vi "Controller Generate Filter Coefficients From Transfer Function.vi"(0 "numerator":dbl[](array[numeric]), 1 "iwl coeff a":i16=2, 3 "iwl coeff b":i16=2, 5 "denominator":dbl[](array[numeric]), 9 "wl":i16=20, 11 "Generate FPGA Code?":bool, 12 "Filter Name":string, 14 "Destination Folder":path) -> (4 "coeff b":dbl[](array[numeric]), 6 "coeff a":dbl[](array[numeric]), 8 "gain":dbl)   [LabVIEW 2011, in "Controller VIs.lvlib"]
uses:
  Controller VIs.lvlib
  <vilib>/addons/Digital Filter Design/_Objects.llb/DFD Output Iwl Obj.ctl
  <vilib>/addons/Digital Filter Design/_Objects.llb/DFD Quantization Settings.ctl
  <vilib>/addons/Digital Filter Design/_Objects.llb/DFD Quantization Sources.ctl
  <vilib>/addons/Digital Filter Design/_Objects.llb/DFD Coef Norm Type.ctl
  <vilib>/addons/Digital Filter Design/_Objects.llb/DFD Phase Setting.ctl
  <vilib>/addons/Digital Filter Design/FXPModel.llb/DFD FXP Quantize Coef (Advanced).vi
  <vilib>/addons/Digital Filter Design/NI_DigFilterLicensed.lvlib
  <vilib>/addons/Digital Filter Design/CodeGen.llb/DFD FXP LabVIEW FPGA Code Generator.vi
panel:
  in  "Error Graph?":bool
  out "phase (deg)":cluster{"Y":dbl[], "Y":dbl[]}[](graph)
  out "gain (dB)":cluster{"Y":dbl[], "Y":dbl[]}[](graph)
  out "max gain error (dB)":dbl
  out "max phase error (deg)":dbl
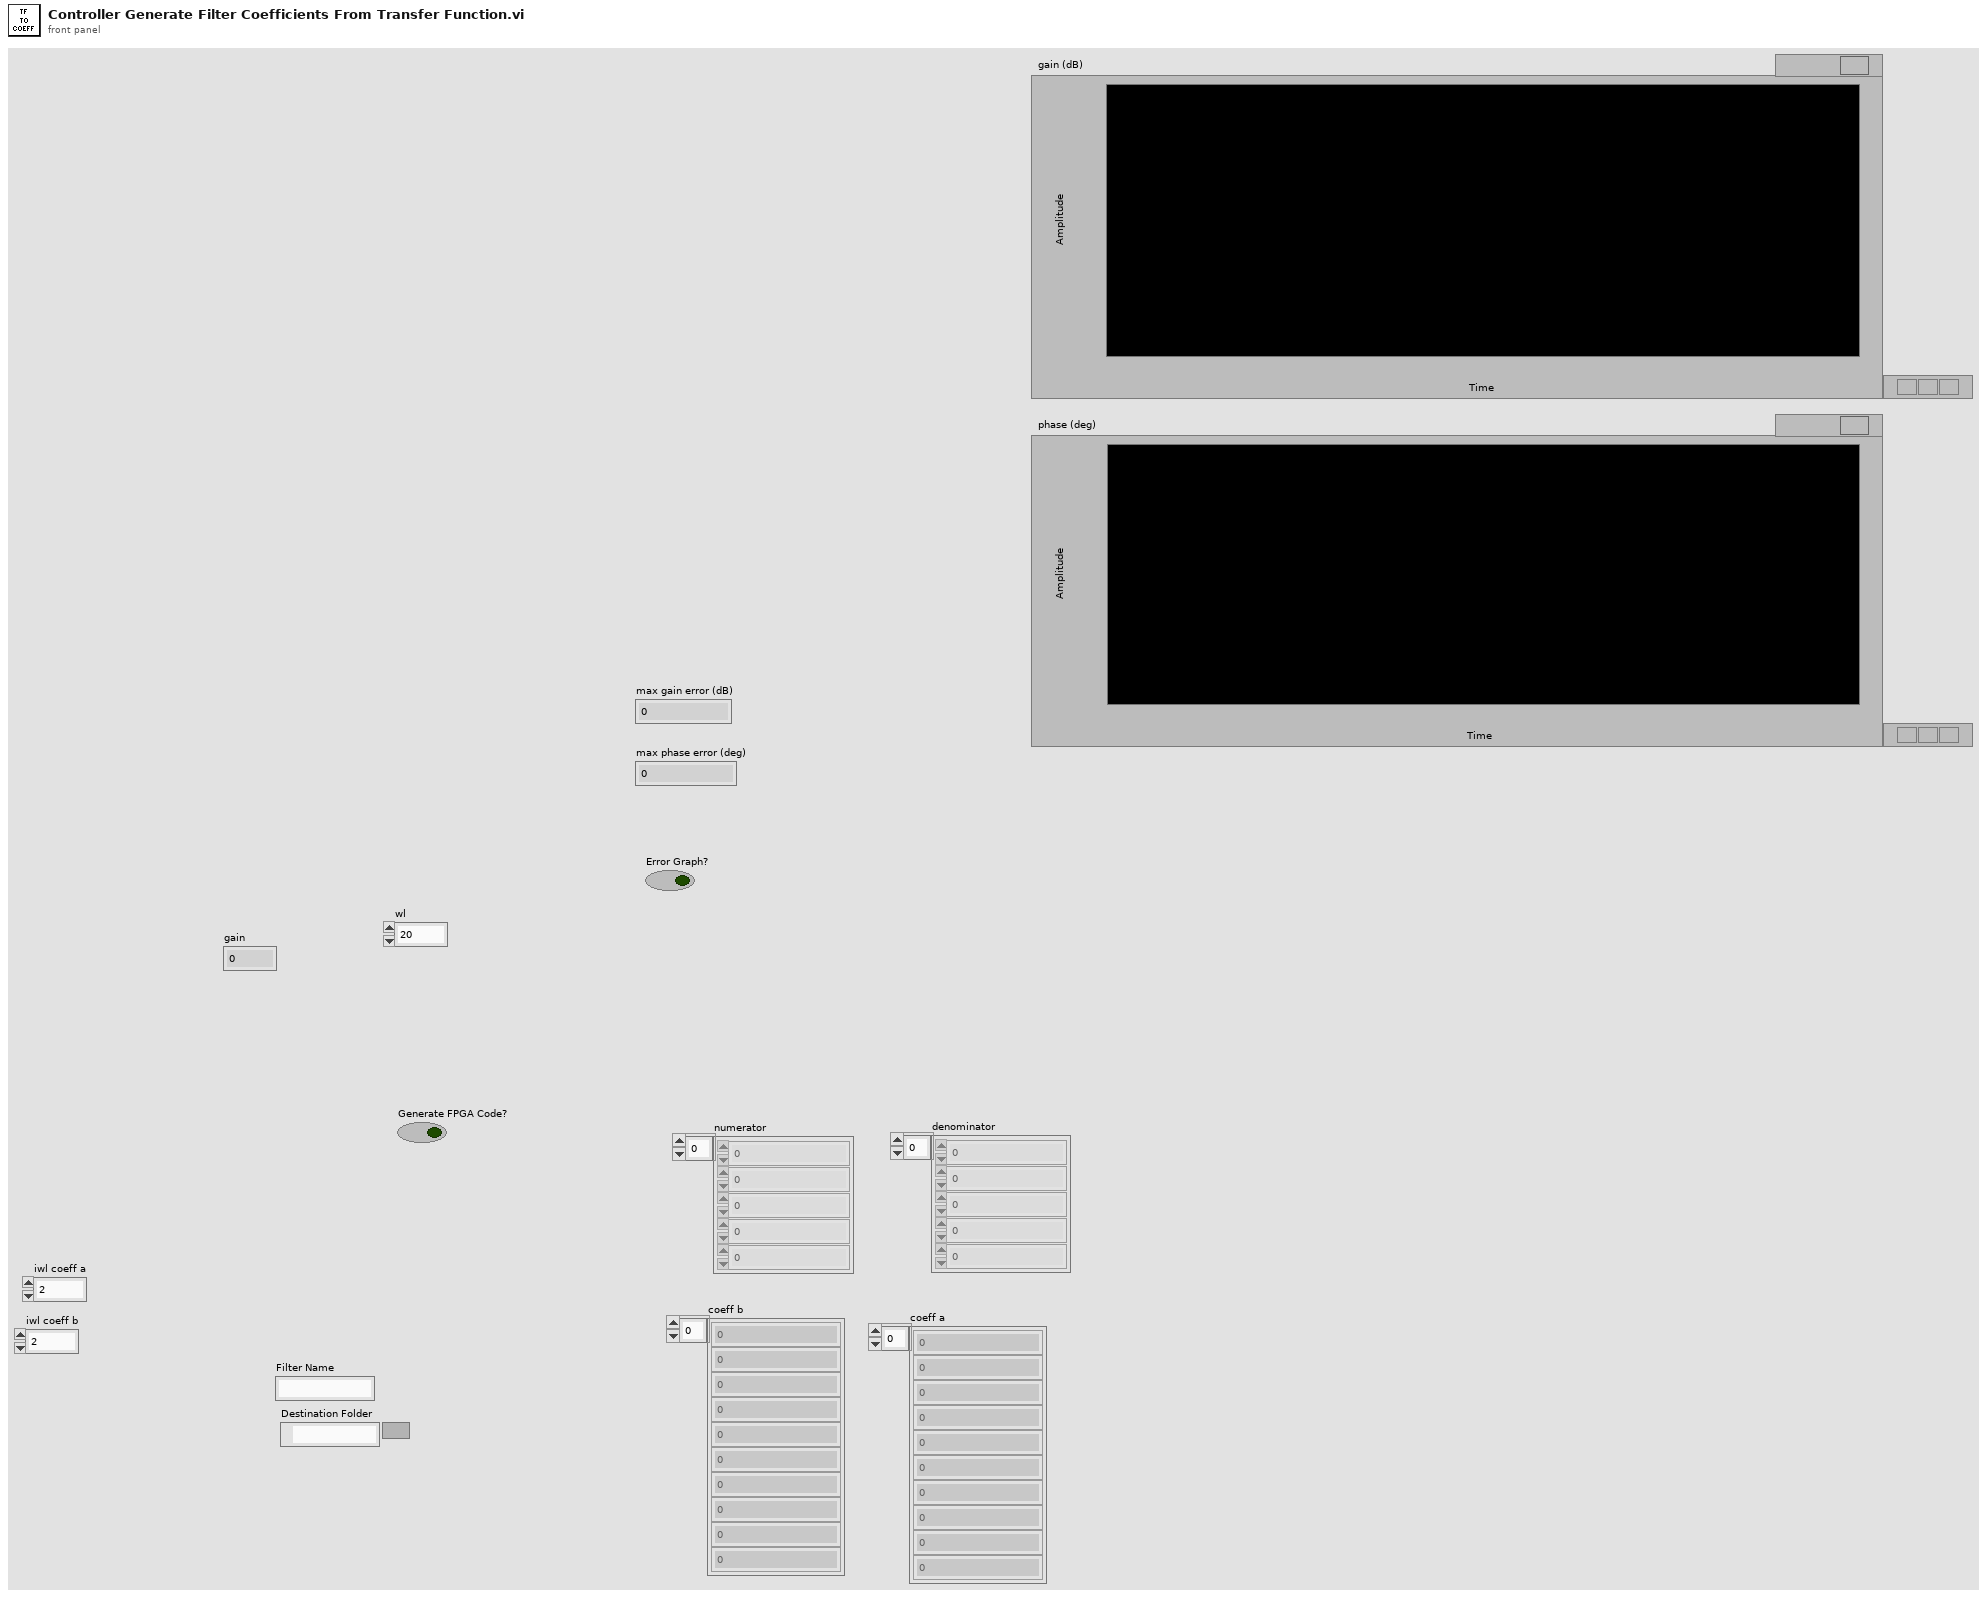
[diagram p1: front panel]
types:
  T1 = typedef "NI_DigFilterLicensed.lvlib/DFD Phase Setting.ctl" = cluster{"unwrap? (F)":bool, "degree? (F)":bool}
  T2 = typedef "NI_DigFilterLicensed.lvlib/DFD Coef Norm Type.ctl" = enum16{"No Norm", "Time Domain 1-Norm", "Time Domain 2-Norm", "Time Domain Inf-Norm"}
  T3 = typedef "NI_DigFilterLicensed.lvlib/DFD Quantization Settings.ctl" = cluster{"source":T4, "wl":i16, "iwl":i16, "overflow mode":enum16{"Saturation", "Wrap"}, "rounding mode":enum16{"Nearest", "Truncation"}, "signed?":bool}
  T4 = typedef "NI_DigFilterLicensed.lvlib/DFD Quantization Sources.ctl" = u16
  T5 = typedef "NI_DigFilterLicensed.lvlib/DFD Output Iwl Obj.ctl" = cluster{"output option":enum16{"Auto", "Same As Input", "User Defined"}, "integer word length":i16}
  T6 = typedef "NI_DigFilterLicensed.lvlib/DFD Filter Obj.ctl" = cluster{"mSRate_Fs":dbl, "mSRate_Version":string, "mSRate_Comments":string, "mSRate_OrgCoef":T7, "mSRate_CurCoef":T7, "mSRate_Quantized?":bool, "mSRate_QCoef":T7, "mSRate_QSettings":T9[], "mSRate_Order":i32, "mSRate_Scaling":cluster{"mSRate_ScaleByPowerOf2?":bool, "mSRate_ScaleType":T2}}
  T7 = typedef "NI_DigFilterLicensed.lvlib/DFD Filter Coef.ctl" = cluster{"type":T8, "gain":dbl, "coef a (k)":dbl[], "coef b (v)":dbl[]}
  T8 = typedef "NI_DigFilterLicensed.lvlib/DFD Filter Structure Type Selector.ctl" = enum16{"Undefined", "FIR Direct Form", "FIR Direct Form Transposed", "FIR Symmetric", "FIR Antisymmetric", "IIR Direct Form I", "IIR Direct Form I Transposed", "IIR Direct Form II", "IIR Direct Form II Transposed", "IIR Cascaded Second Order Sections Form I", "IIR Cascaded Second Order Sections Form I Transposed", "IIR Cascaded Second Order Sections Form II", "IIR Cascaded Second Order Sections Form II Transposed", "Lattice Allpass (basic sections)", "Lattice Allpass (one multiplier sections)", "Lattice Allpass (normalized sections)", "Lattice AR (basic sections)", "Lattice AR (one multiplier sections)", "Lattice AR (normalized sections)", "Lattice MA (minimum phase)", "Lattice MA (maximum phase)", "Lattice ARMA (basic sections)", "Lattice ARMA (one multiplier sections)", "Lattice ARMA (normalized sections)"}
  T9 = typedef "NI_DigFilterLicensed.lvlib/dfd_Internal Quantization Settings.ctl" = cluster{"source":T10, "wl":i16, "iwl":i16, "overflow mode":enum16{"Saturation", "Wrap"}, "rounding mode":enum16{"Nearest", "Truncation"}, "signed?":bool}
  T10 = typedef "NI_DigFilterLicensed.lvlib/dfd_Internal Quantization Srcs.ctl" = u16
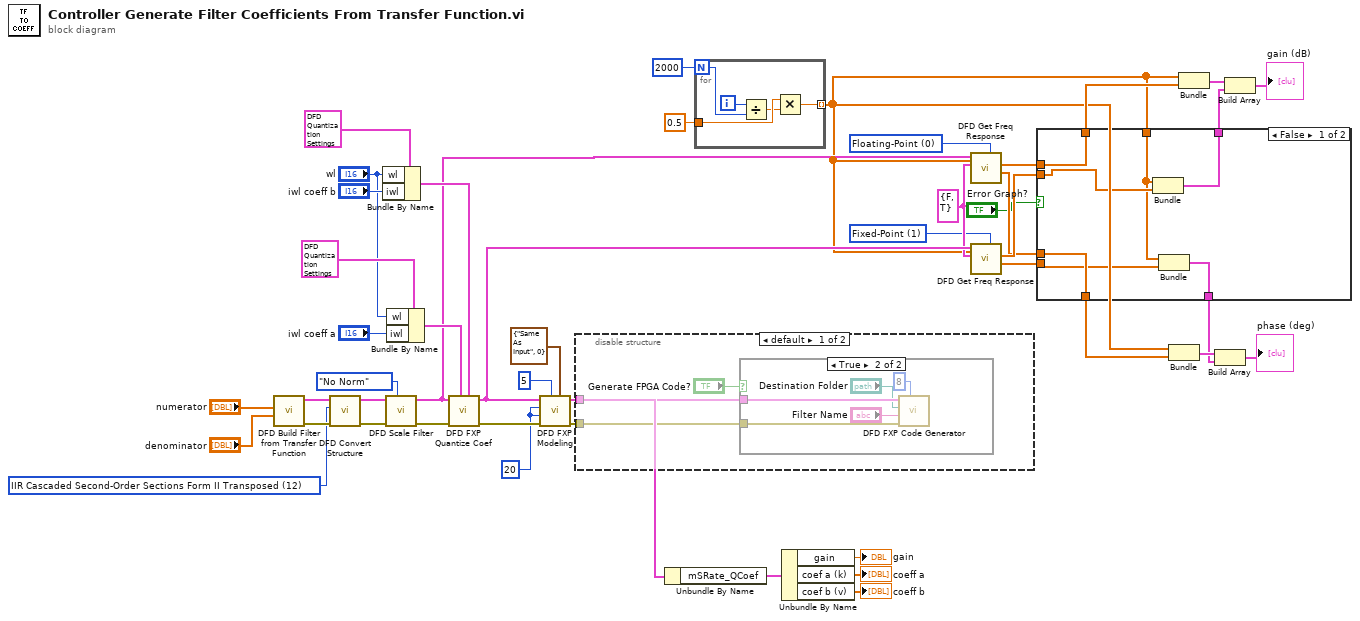
[diagram p0: block diagram]
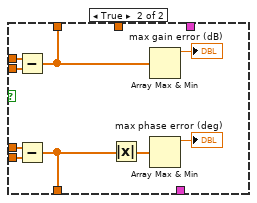
[diagram p4: hidden frame]
diagram:
  w20 = T1 {"unwrap? (F)"=FALSE, "degree? (F)"=TRUE} ("phase view")
  w17 = u16 0 items=["Floating-Point", "Fixed-Point"] ("output option")
  w19 = u16 1 items=["Floating-Point", "Fixed-Point"] ("output option")
  w38 = i16 20 ("input word length")
  w45 = u16 12 items=["FIR Direct Form"=1, "FIR Direct Form Transposed"=2, "FIR Symmetric"=3, "FIR Antisymmetric"=4, "IIR Direct Form I"=5, "IIR Direct Form I Transposed"=6, "IIR Direct Form II"=7, "IIR Direct Form II Transposed"=8, "IIR Cascaded Second-Order Sections Form I"=9, "IIR Cascaded Second-Order Sections Form I Transposed"=10, "IIR Cascaded Second-Order Sections Form II"=11, "IIR Cascaded Second-Order Sections Form II Transposed"=12, "Lattice Allpass (basic sections)"=13, "Lattice Allpass (one multiplier sections)"=14, "Lattice Allpass (normalized sections)"=15, "Lattice AR (basic sections)"=16, "Lattice AR (one multiplier sections)"=17, "Lattice AR (normalized sections)"=18, "Lattice MA (minimum phase)"=19, "Lattice MA (maximum phase)"=20, "Lattice ARMA (basic sections)"=21, "Lattice ARMA (one multiplier sections)"=22, "Lattice ARMA (normalized sections)"=23] ("target structure")
  n1 = call <vilib>:"DFD Build Filter from Transfer Function.vi"("denominator"="denominator", "numerator"="numerator") -> ("error out"=w46:errorcluster, "filter out"=w40:T6)  [unwired: 8 in]
  n2 = call <vilib>:"DFD Convert Structure.vi"("error in (no error)"=w46, "target structure"=w45, "filter in"=w40) -> ("error out"=w27:errorcluster, "filter out"=w28:T6)  [unwired: 7 in]
  n3 = Bundle By Name(cluster=T3 {"source"=7, "wl"=20, "iwl"=1, "overflow mode"=enum."Saturation", "rounding mode"=enum."Nearest", "signed?"=TRUE} ("coefficients b/v quantizer"), "wl"="wl", "iwl"="iwl coeff b") -> (w31:T3)
  n4 = call <vilib>:"DFD Scale Filter.vi"("scale type"=DFD_Coef_Norm_Type."No Norm", "error in (no error)"=w27, "filter in"=w28) -> ("error out"=w26:errorcluster, "filter out"=w22:T6)  [unwired: 7 in]
  n5 = Bundle By Name(cluster=T3 {"source"=0, "wl"=20, "iwl"=1, "overflow mode"=enum."Saturation", "rounding mode"=enum."Nearest", "signed?"=TRUE} ("coefficients a/k quantizer"), "wl"="wl", "iwl"="iwl coeff a") -> (w30:T3)
  n6 = call-poly <vilib>:"DFD FXP Quantize Coef.vi"("coefficients b/v quantizer"=w31, "coefficients a/k quantizer"=w30, "error in (no error)"=w26, "filter in"=w22) -> ("error out"=w44:errorcluster, "filter out"=w21:T6)  [unwired: 6 in]
  n7 = call <vilib>:"DFD FXP Modeling.vi"("output integer word length"=T5 {"output option"=enum."Same As Input", "integer word length"=0}, "input integer word length"=i16 5, "error in (no error)"=w44, "output word length"=w38, "input word length"=w38, "filter in"=w21) -> ("error out"=w47:errorcluster, "filter out"=w36:T6)  [unwired: 4 in]
  n8 = disable-structure shown="default" {
    disable-tunnel: w47 -> [w50 _]
    disable-tunnel: w36 -> [w49 _]
    frame condition #0 {
      n9 = case shown="True" "Generate FPGA Code?" {
        tunnel: w50 -> [_ w55]
        tunnel: w49 -> [_ w54]
        frame False {
        }
        frame True {
          n10 = call-poly <vilib>:"DFD FXP Code Generator.vi"("# channels"=8, "error in (no error)"=w55, "filter name"="Filter Name", "destination folder"="Destination Folder", "filter in"=w54) -> ()  [unwired: 2 in, 5 out]
        }
      }
    }
    frame condition #1 (active) {
    }
  }
  n11 = Unbundle By Name(w36) -> ("mSRate_QCoef"=w43:T7)
  n12 = for {
    N: 2000 -> [w59]
    tunnel: 0.5 -> [w58]
    tunnel: [w56] -> w4 mode=indexing
    i -> [w60]
    n13 = Divide(x=w60, y=w59) -> (x/y=w57:dbl)
    n14 = Multiply(x=w58, y=w57) -> (x*y=w56:dbl)
  }
  n15 = Unbundle By Name(w43) -> ("gain"=→"gain":dbl, "coef a (k)"=→"coeff a":dbl[], "coef b (v)"=→"coeff b":dbl[])
  n16 = call <vilib>:"DFD Get Freq Response.vi"("output option"=w17, "freq points [Hz]"=w4, "phase view"=w20, "filter in"=w22) -> ("phase"=w14:dbl[], "magnitude"=w16:dbl[])  [unwired: 4 in, 2 out]
  n17 = call <vilib>:"DFD Get Freq Response.vi"("output option"=w19, "freq points [Hz]"=w4, "phase view"=w20, "filter in"=w21) -> ("phase"=w13:dbl[], "magnitude"=w15:dbl[])  [unwired: 4 in, 2 out]
  n18 = case shown="False" "Error Graph?" {
    tunnel: w16 -> [w67 w76]
    tunnel: w15 -> [w65 w75]
    tunnel: w14 -> [w66 w74]
    tunnel: w13 -> [w62 w73]
    tunnel: [w67 w68] -> w11
    tunnel: [w66 w69] -> w6
    tunnel: w4 -> [w63 _]
    tunnel: [w64 _] -> w3
    tunnel: [w61 _] -> w2
    frame False {
      n19 = Bundle(w63, "magnitude"=w65) -> (w64:cluster{dbl[], "magnitude":dbl[]})  [unwired: 1 in]
      n20 = Bundle(w63, "phase"=w62) -> (w61:cluster{dbl[], "phase":dbl[]})  [unwired: 1 in]
    }
    frame True {
      n21 = Subtract(x=w76, y=w75) -> (x-y=w68:dbl[])
      n22 = Subtract(x=w74, y=w73) -> (x-y=w69:dbl[])
      n23 = Absolute Value(x=w69) -> (abs(x)=w72:dbl[])
      n24 = Array Max & Min(array=w68) -> (max value=→"max gain error (dB)":dbl)  [unwired: 3 out]
      n25 = Array Max & Min(array=w72) -> (max value=→"max phase error (deg)":dbl)  [unwired: 3 out]
    }
  }
  n26 = Bundle(w4, "phase"=w6) -> (w7:cluster{dbl[], "phase":dbl[]})  [unwired: 1 in]
  n27 = Bundle(w4, "magnitude"=w11) -> (w10:cluster{dbl[], "magnitude":dbl[]})  [unwired: 1 in]
  n28 = Build Array(w7, w2) -> (→"phase (deg)":cluster{dbl[], "phase":dbl[]}[])
  n29 = Build Array(w10, w3) -> (→"gain (dB)":cluster{dbl[], "magnitude":dbl[]}[])
